vi "Configure.vi"(8 "error in (no error)":errorcluster, 11 "Build Package Item in":refnum<class "Build Package Item.lvclass">) -> (0 "error out":errorcluster, 3 "Build Package Item out":refnum<class "Build Package Item.lvclass">)   [LabVIEW 2019, in "VIPM.lvlib" / "Build Package Item.lvclass"]
uses:
  Build Package Item.lvclass
  Build Package Item.lvclass/Build Package Item.ctl
panel:
  in  "Build Specification":path
  in  "OK":bool
  in  "Cancel":bool
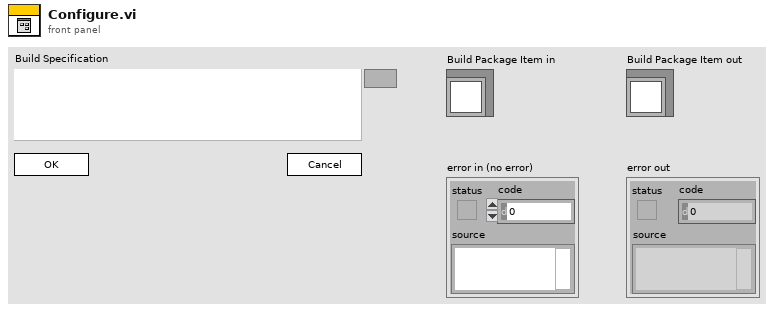
[diagram p1: front panel]
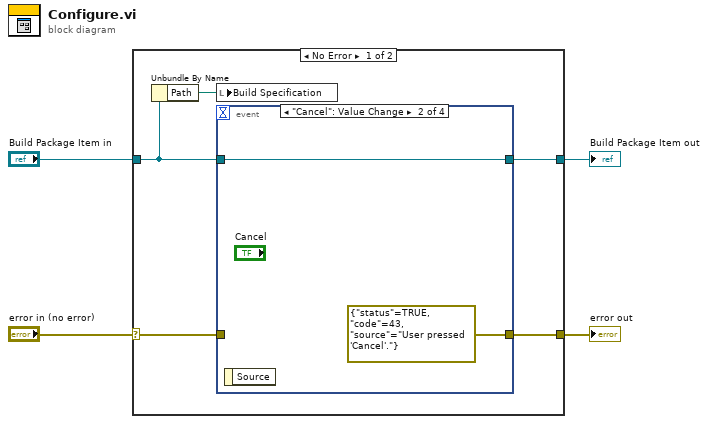
[diagram p0: block diagram]
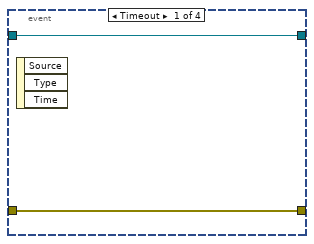
[diagram p2: hidden frame]
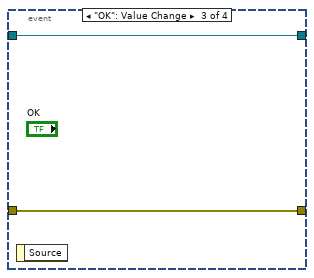
[diagram p3: hidden frame]
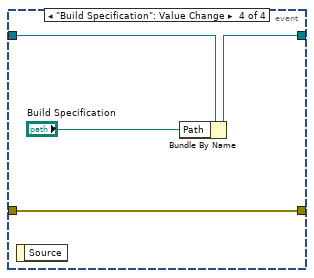
[diagram p4: hidden frame]
diagram:
  n1 = case shown="No Error" "error in (no error)" {
    selector: "error in (no error)" -> [w5 w21]
    tunnel: [w6 w21] -> w3
    tunnel: [w9 w20] -> w1
    tunnel: "Build Package Item in" -> [w8 w20]
    frame No Error {
      n2 = Unbundle By Name(w8) -> ("Path"=w7:path)
      n3 = local write "Build Specification"(w7) -> ()
      n4 = event shown="[1] \"Cancel\": Value Change" {
        selector: _ -> [_ _ _ _]
        dyn-events: _ -> [_ _ _ _]
        timeout: _ -> [_ _ _ _]
        tunnel: w8 -> [w11 w13 w15 w19]
        tunnel: [w11 w13 w15 w18] -> w9
        tunnel: [w10 errorcluster {"status"=TRUE, "code"=43, "source"="User pressed 'Cancel'."} ("error in (no error)") w14 w16] -> w6
        tunnel: w5 -> [w10 _ w14 w16]
        event Timeout {
          n5 = event-data() -> ()  [unwired: 1 in, 3 out]
        }
        event "Cancel": Value Change {
          n6 = event-data() -> ()  [unwired: 1 in, 1 out]
        }
        event "OK": Value Change {
          n7 = event-data() -> ()  [unwired: 1 in, 1 out]
        }
        event "Build Specification": Value Change {
          n8 = event-data() -> ()  [unwired: 1 in, 1 out]
          n9 = Bundle By Name(cluster=w19, "Path"="Build Specification") -> (w18:refnum<class "Build Package Item.lvclass">)
        }
      }
    }
    frame Error {
    }
  }
  "error out" <- w3
  "Build Package Item out" <- w1
